vi "4-2-2 read & parsing JSON.vi"(8 "sensor_data":T1={"temp_reactor"=81.27072750007478, "temp_coolant"=91.17736124894773, "press_reactor"=73.46732895466137, "stir_speed"=81.53437024634668, "coolant_flow"=TRUE, "exhaust_valve"=FALSE, "timestamp"="21:38:10"}, 11 "read JSON data":string) -> (3 "sensor_data out":T1)   [LabVIEW 2020]
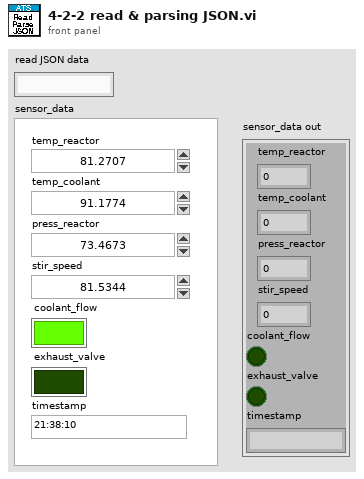
[diagram p1: front panel]
types:
  T1 = cluster{"temp_reactor":dbl, "temp_coolant":dbl, "press_reactor":dbl, "stir_speed":dbl, "coolant_flow":bool, "exhaust_valve":bool, "timestamp":string}
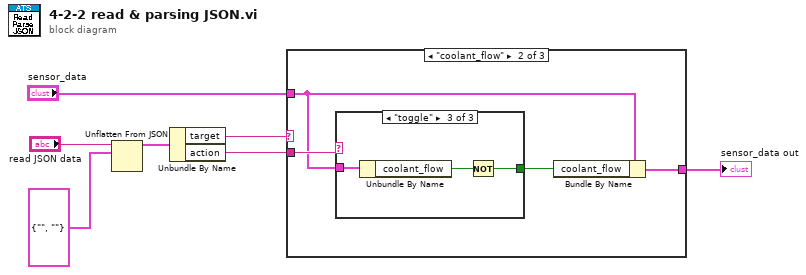
[diagram p0: block diagram]
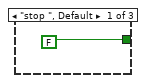
[diagram p3: hidden frame]
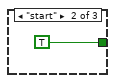
[diagram p4: hidden frame]
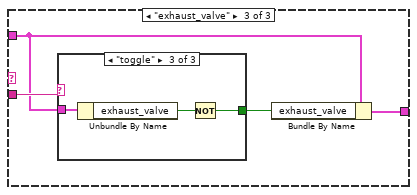
[diagram p5: hidden frame]
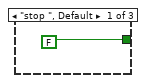
[diagram p6: hidden frame]
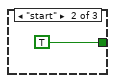
[diagram p7: hidden frame]
diagram:
  n1 = Unflatten From JSON(JSON string="read JSON data", type and defaults=cluster{"target":string, "action":string} {"target"="", "action"=""}) -> (value=w5:cluster{"target":string, "action":string})  [unwired: 5 in, 1 out]
  n2 = Unbundle By Name(w5) -> ("target"=w4:string, "action"=w3:string)
  n3 = case shown="\"coolant_flow\"" w4 {
    tunnel: w3 -> [_ w12 w21]
    tunnel: "sensor_data" -> [w8 w10 w19]
    tunnel: [w8 w9 w18] -> w1
    frame "", Default {
    }
    frame "coolant_flow" {
      n4 = case shown="\"toggle\"" w12 {
        tunnel: [FALSE TRUE w15] -> w11
        tunnel: w10 -> [_ _ w17]
        frame "stop ", Default {
        }
        frame "start" {
        }
        frame "toggle" {
          n5 = Unbundle By Name(w17) -> ("coolant_flow"=w16:bool)
          n6 = Not(x=w16) -> (.not. x?=w15:bool)
        }
      }
      n7 = Bundle By Name(cluster=w10, "coolant_flow"=w11) -> (w9:T1)
    }
    frame "exhaust_valve" {
      n8 = case shown="\"toggle\"" w21 {
        tunnel: [FALSE TRUE w24] -> w20
        tunnel: w19 -> [_ _ w26]
        frame "stop ", Default {
        }
        frame "start" {
        }
        frame "toggle" {
          n9 = Unbundle By Name(w26) -> ("exhaust_valve"=w25:bool)
          n10 = Not(x=w25) -> (.not. x?=w24:bool)
        }
      }
      n11 = Bundle By Name(cluster=w19, "exhaust_valve"=w20) -> (w18:T1)
    }
  }
  "sensor_data out" <- w1
